vi "SSCP_configureDevice.vi"(2 "error in (no error)":errorcluster, 3 "Device Configuration in":T1={"Device name"="default", "Device number"="0", "Serial Port"="COM9", "Serial baud rate"="115200", "Base Port"="3000", "Device Serial Number"="0", "Interface Timeout"="10000", "Interface Type"=""}) -> (0 "error out":errorcluster, 1 "Device Configuration out":T1)   [LabVIEW 2020]
uses:
  typedefs/Device Configuration.ctl
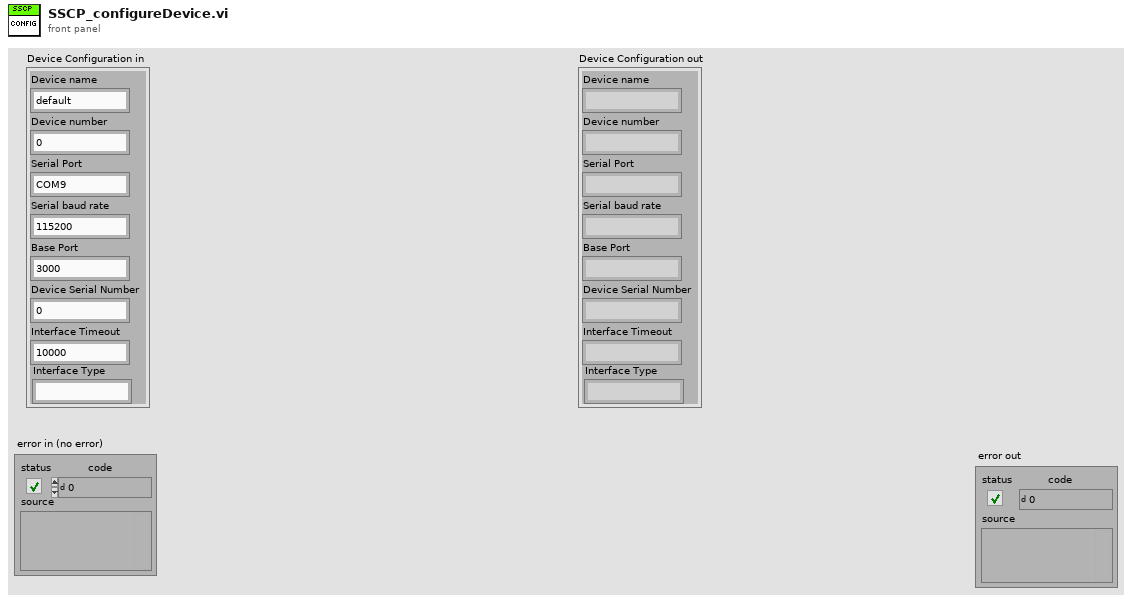
[diagram p1: front panel]
types:
  T1 = typedef "Device Configuration.ctl" = cluster{"Device name":string, "Device number":string, "Serial Port":string, "Serial baud rate":string, "Base Port":string, "Device Serial Number":string, "Interface Timeout":string, "Interface Type":string}
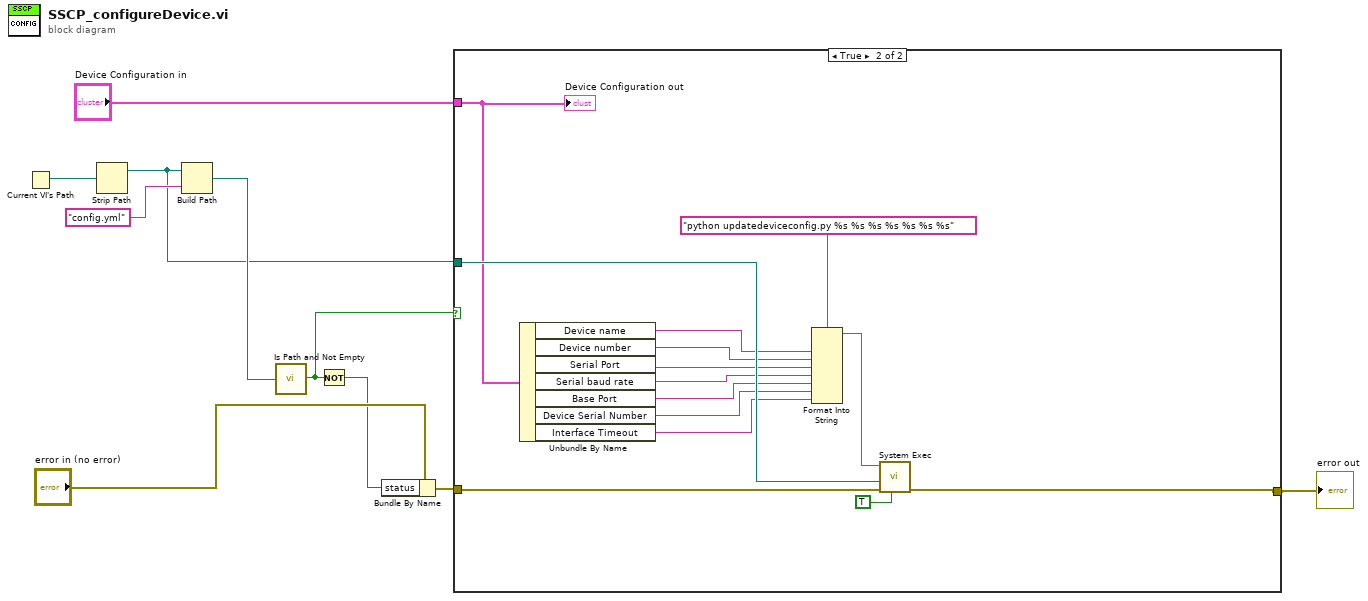
[diagram p0: block diagram]
diagram:
  n1 = Current VI's Path() -> (path=w10:path)
  n2 = Strip Path(path=w10) -> (stripped path=w2:path)  [unwired: 1 out]
  n3 = Build Path(base path=w2, name or relative path="config.yml") -> (appended path=w3:path)
  n4 = call <vilib>:"Is Path and Not Empty.vi"("path"=w3) -> ("Is Path and Not Empty?"=w5:bool)  [unwired: 4 in]
  n5 = Not(x=w5) -> (.not. x?=w7:bool)
  n6 = Bundle By Name(cluster="error in (no error)", "status"=w7) -> (w6:errorcluster)
  n7 = case shown="True" w5 {
    tunnel: w6 -> [w11 w25]
    tunnel: [w11 w20] -> w4
    tunnel: w2 -> [_ w23]
    tunnel: "Device Configuration in" -> [_ w19]
    frame False {
    }
    frame True {
      n8 = Unbundle By Name(w19) -> ("Device name"=w18:string, "Device number"=w17:string, "Serial Port"=w16:string, "Serial baud rate"=w15:string, "Base Port"=w14:string, "Device Serial Number"=w13:string, "Interface Timeout"=w12:string)
      n9 = Format Into String(format string="python updatedeviceconfig.py %s %s %s %s %s %s %s", w18, w17, w16, w15, w14, w13, w12) -> (resulting string=w21:string)  [unwired: 2 in, 1 out]
      n10 = call <vilib>:"System Exec.vi"("run minimized? (F)"=TRUE, "error in (no error)"=w25, "working directory"=w23, "command line"=w21) -> ("error out"=w20:errorcluster)  [unwired: 4 in, 3 out]
      "Device Configuration out" <- w19
    }
  }
  "error out" <- w4
